vi "多参数数据插入.vi"(8 "error in (no error)":errorcluster caption="错误输入（无错误）", 9 "编号":string, 10 "columns enable":T1, 11 "data in":T2) -> (0 "error out":errorcluster)   [LabVIEW 2022 SP3, in "斯坦道多参数.lvlib"]
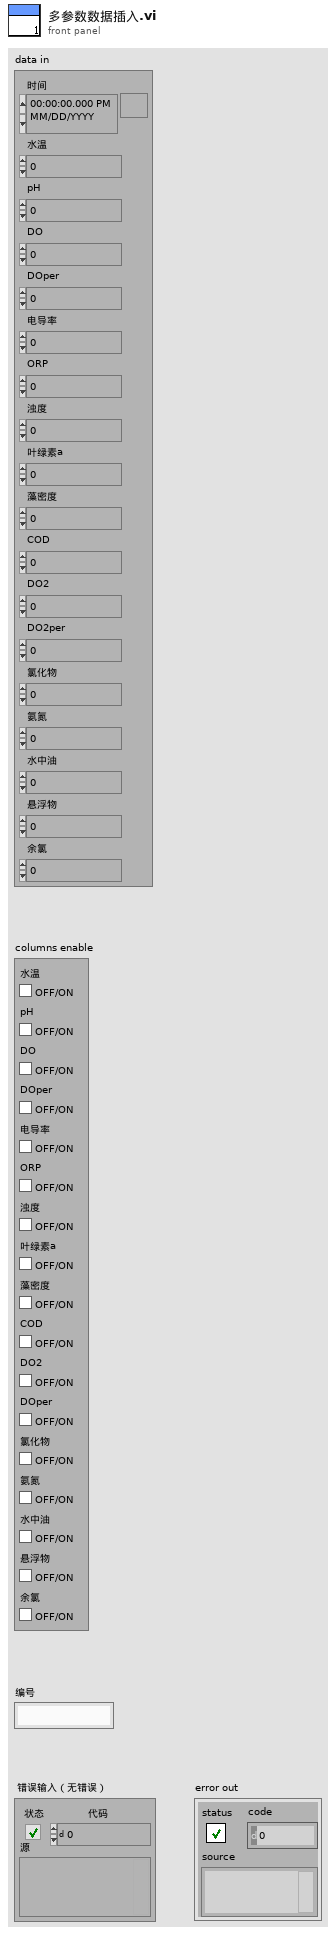
[diagram p1: front panel]
types:
  T1 = cluster{"水温":bool, "pH":bool, "DO":bool, "DOper":bool, "电导率":bool, "ORP":bool, "浊度":bool, "叶绿素a":bool, "藻密度":bool, "COD":bool, "DO2":bool, "DOper":bool, "氯化物":bool, "氨氮":bool, "水中油":bool, "悬浮物":bool, "余氯":bool}
  T2 = cluster{"时间":timestamp, "水温":dbl, "pH":dbl, "DO":dbl, "DOper":dbl, "电导率":dbl, "ORP":dbl, "浊度":dbl, "叶绿素a":dbl, "藻密度":dbl, "COD":dbl, "DO2":dbl, "DO2per":dbl, "氯化物":dbl, "氨氮":dbl, "水中油":dbl, "悬浮物":dbl, "余氯":dbl}
  T3 = cluster{"columns外部输入":bool, "columns input":string[]}
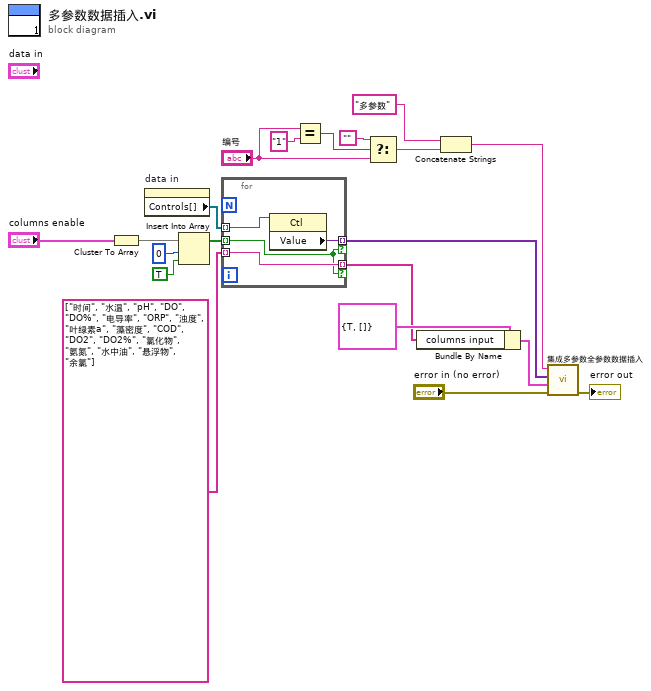
[diagram p0: block diagram]
diagram:
  n1 = Cluster To Array(cluster="columns enable") -> (array=w11:bool[])
  n2 = property on="data in" class="Clust (strict)"() -> ("Controls[]"=w13:refnum<vi>[])  [unwired: 2 in, 2 out]
  n3 = Insert Into Array(array=w11, index=0 ("索引"), new element=TRUE ("新元素/子数组")) -> (w12:bool[])
  n4 = for {
    tunnel: w13 -> [w24] mode=indexing
    tunnel: [w23] -> w6 mode=indexing if=w21
    tunnel: string[] ["时间", "水温", "pH", "DO", "DO%", "电导率", "ORP", "浊度", "叶绿素a", "藻密度", "COD", "DO2", "DO2%", "氯化物", "氨氮", "水中油", "悬浮物", "余氯"] -> [w22] mode=indexing
    tunnel: [w22] -> w1 mode=indexing if=w21
    tunnel: w12 -> [w21] mode=indexing
    n5 = property class="Ctl"(reference=w24) -> ("Value"=w23:variant)  [unwired: 1 in, 2 out]
  }
  n6 = Equal?(x="编号", y="1") -> (x = y?=w17:bool)
  n7 = Select(t="", s=w17, f="编号") -> (s? t:f=w14:string)
  n8 = Bundle By Name(cluster=T3 {"columns外部输入"=TRUE, "columns input"=[]} ("columns外部输入"), "columns input"=w1) -> (w2:T3)
  n9 = Concatenate Strings("多参数" ("字符串"), w14) -> (w5:string)
  n10 = call "集成多参数全参数数据插入.vi"("Tabe Name"=w5, "data"=w6, "columns外部输入"=w2, "错误输入（无错误）"="error in (no error)") -> ("错误输出"=→"error out":errorcluster)  [unwired: 6 in]
